vi "traingleDet.vi"(8 "error in (no error)":errorcluster, 11 "Image":T1) -> (0 "error out":errorcluster, 2 "Number of Matches":i32, 3 "Matches (pixel)":T2(array[cluster]) {"Bounding Box"."y" format="%.2f"; "Bounding Box"."x" format="%.2f"; "Score" format="%.2f"; "Scale" format="%.2f"; "Angle" format="%.2f"; "Position"."y" format="%.2f"; "Position"."x" format="%.2f"})   [LabVIEW 2023]
uses:
  <vilib>/vision/Image Controls.llb/IMAQ Image.ctl
  <vilib>/vision/NI_Vision_Development_Module.lvlib
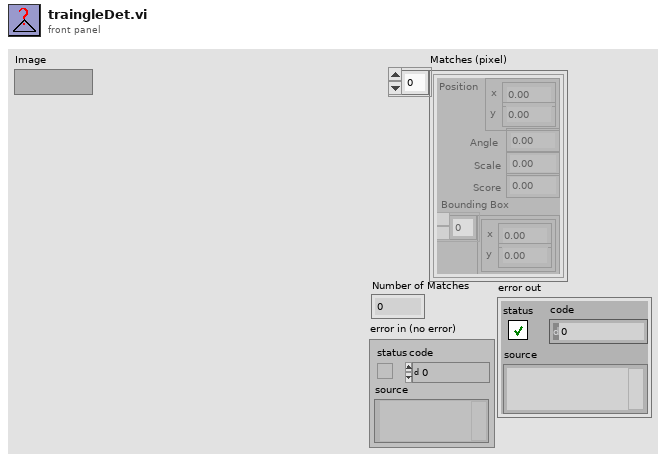
[diagram p1: front panel]
types:
  T1 = typedef "IMAQ Image.ctl" = refnum<image>
  T2 = cluster{"Position":cluster{"x":sgl, "y":sgl}, "Angle":sgl, "Scale":sgl, "Score":sgl, "Bounding Box":cluster{"x":sgl, "y":sgl}[]}[]
  T3 = cluster{"Number of Matches Requested":i32, "Minimum Match Score":sgl, "Angle Ranges":cluster{"Start Angle":sgl, "End Angle":sgl}[]}
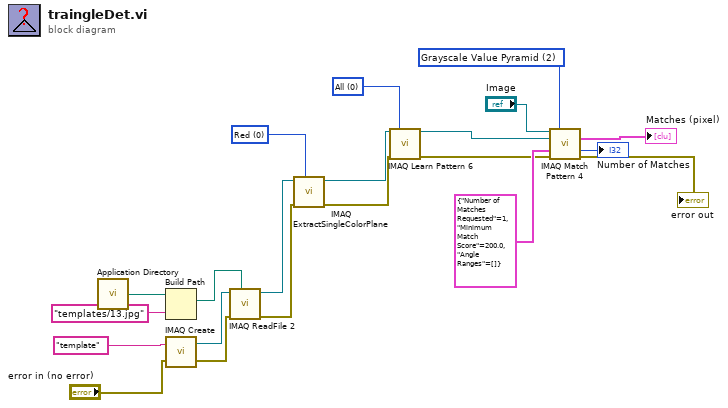
[diagram p0: block diagram]
diagram:
  w9 = 2 items=["All", "Low Discrepancy Sampling", "Grayscale Value Pyramid", "Gradients Pyramid"] ("Algorithm")
  w12 = 0 items=["Red", "Green", "Blue", "Hue", "Saturation", "Luminance", "Value", "Intensity"] ("Color Plane")
  w21 = 0 items=["All", "Low Discrepancy Sampling", "Grayscale Value Pyramid", "Gradients Pyramid"] ("Algorithm")
  n1 = call <vilib>:"Application Directory.vi"() -> ("Application Directory"=w17:path)
  n2 = Build Path(base path=w17, name or relative path="templates/13.jpg") -> (appended path=w15:path)
  n3 = call "IMAQ Create"("Image Name"="template" ("name or relative path"), "error in (no error)"="error in (no error)") -> ("New Image"=w14:T1, "error out"=w4:errorcluster)  [unwired: 3 in]
  n4 = call "IMAQ ReadFile 2"("File Path"=w15, "error in (no error)"=w4, "Image"=w14) -> ("error out"=w3:errorcluster, "Image Out"=w11:T1)  [unwired: 4 in, 3 out]
  n5 = call "IMAQ ExtractSingleColorPlane"("Color Plane"=w12, "error in (no error)"=w3, "Image Src"=w11) -> ("error out"=w2:errorcluster, "Image Dst Out"=w10:T1)  [unwired: 7 in]
  n6 = call "IMAQ Learn Pattern 6"("Image"=w10, "Algorithm"=w21, "error in (no error)"=w2) -> ("Template Image Out"=w20:T1, "error out"=w1:errorcluster)  [unwired: 10 in, 1 out]
  n7 = call "IMAQ Match Pattern 4"("Image"="Image", "Algorithm"=w9, "Template Image"=w20, "Parameters"=T3 {"Number of Matches Requested"=1, "Minimum Match Score"=200.0, "Angle Ranges"=[]}, "error in (no error)"=w1) -> ("Matches (pixel)"=→"Matches (pixel)":T2, "Number of Matches"=→"Number of Matches":i32, "error out"=→"error out":errorcluster)  [unwired: 6 in, 2 out]
